vi "Get System Name.vi"(8 "error in (no error)":errorcluster, 11 "Forward Drive in":refnum<class "Forward Drive.lvclass">) -> (0 "error out":errorcluster, 2 "System Name":string, 3 "Forward Drive out":refnum<class "Forward Drive.lvclass">)   [LabVIEW 2014, in "Forward Drive.lvlib" / "Forward Drive.lvclass"]
uses:
  Forward Drive.lvclass
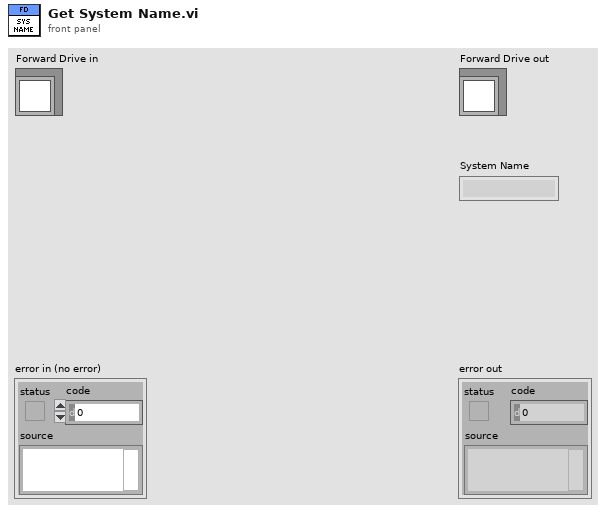
[diagram p1: front panel]
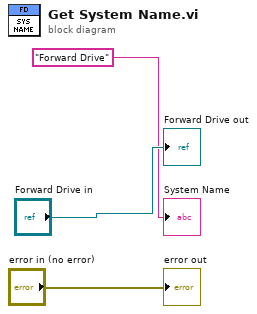
[diagram p0: block diagram]
diagram:
  "error out" <- "error in (no error)"
  "Forward Drive out" <- "Forward Drive in"
  "System Name" <- "Forward Drive"
